vi "GetDVR.vi"(8 "error in (no error)":errorcluster, 11 "Shadow in":refnum<class "Shadow.lvclass">) -> (0 "error out":errorcluster, 2 "DVR":refnum<data-value>, 3 "Shadow out":refnum<class "Shadow.lvclass">)   [LabVIEW 2021, in "UIShadow.lvlib" / "Shadow.lvclass"]
uses:
  Shadow.lvclass
  Data.ctl
  Shadow.lvclass/Shadow.ctl
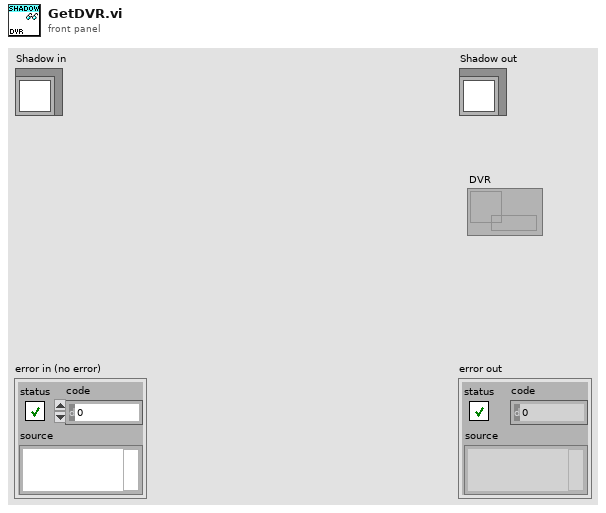
[diagram p1: front panel]
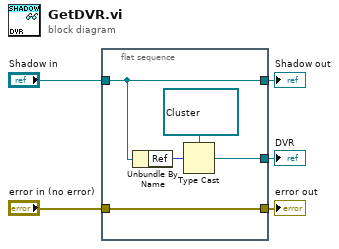
[diagram p0: block diagram]
diagram:
  n1 = flat-sequence {
    tunnel: [w8] -> w5
    tunnel: "Shadow in" -> [w6]
    tunnel: "error in (no error)" -> [w7]
    tunnel: [w7] -> w3
    tunnel: [w6] -> w1
    frame #0 {
      n2 = Unbundle By Name(w6) -> ("Ref"=w10:u64)
      n3 = Type Cast(type=refnum<data-value> refnum ("data value reference"), x=w10) -> (*(type *) &x=w8:refnum<data-value>)
    }
  }
  "error out" <- w3
  "Shadow out" <- w1
  "DVR" <- w5
